vi "ex 3.vi"() -> ()   [LabVIEW 2019]
panel:
  out "Array":i32[](array[numeric])
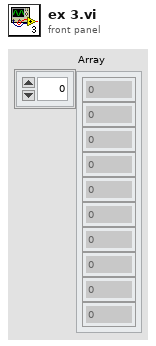
[diagram p1: front panel]
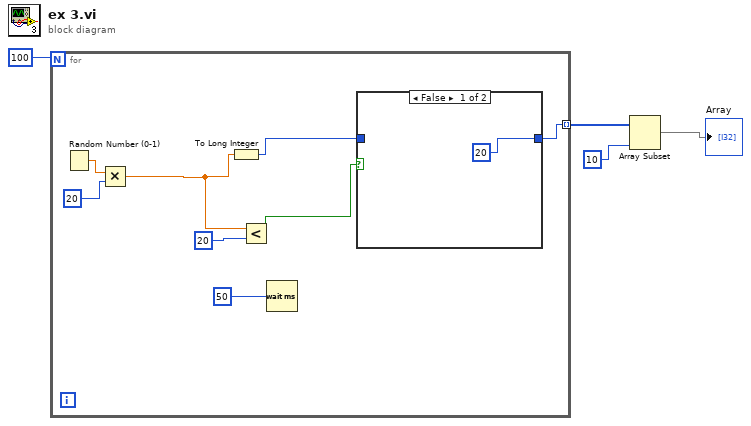
[diagram p0: block diagram]
diagram:
  n1 = for {
    N: 100 -> [_]
    tunnel: [w9] -> w2 mode=indexing
    n2 = Random Number (0-1)() -> (number: 0 to 1=w12:dbl)
    n3 = Multiply(x=w12, y=20) -> (x*y=w5:dbl)
    n4 = To Long Integer(number=w5) -> (32bit integer=w8:i32)
    n5 = Less?(x=w5, y=20) -> (x < y?=w6:bool)
    n6 = Wait (ms)(milliseconds to wait=50) -> ()  [unwired: 1 out]
    n7 = case shown="False" w6 {
      tunnel: [20 w14] -> w9
      tunnel: w8 -> [_ w14]
      frame False {
      }
      frame True {
      }
    }
  }
  n8 = Array Subset(array=w2, length=10) -> (→"Array":i32[])  [unwired: 1 in]
